vi "Main.vi"() -> ()   [LabVIEW 2020]
panel:
  in  "Test Execution":bool caption="Lab Manager"
  in  "Test Engineering":bool caption="Lab Manager"
  in  "Lab Manager":bool
  # "Please select your operation"
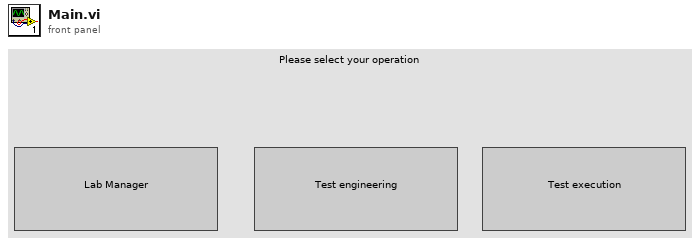
[diagram p1: front panel]
types:
  T1 = enum32{"Invalid", "Standard", "Closed", "Hidden", "Minimized", "Maximized"}
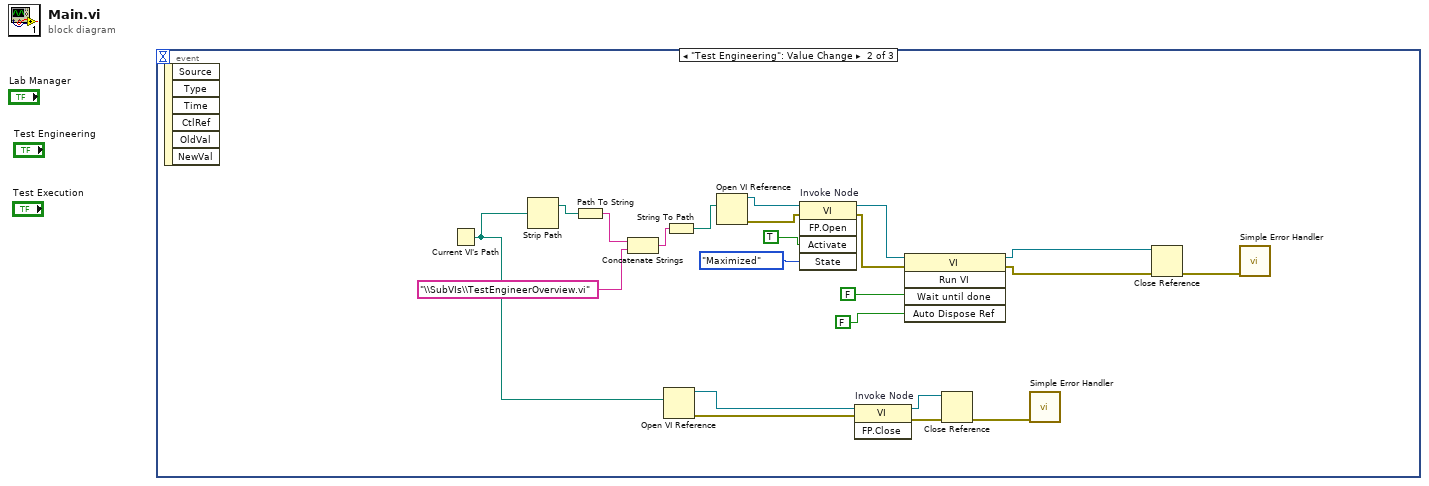
[diagram p0: block diagram]
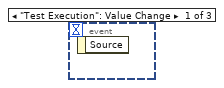
[diagram p2: hidden frame]
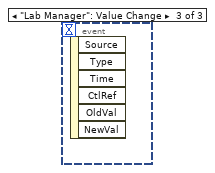
[diagram p3: hidden frame]
diagram:
  n1 = event shown="[1] \"Test Engineering\": Value Change" {
    selector: _ -> [_ _ _]
    dyn-events: _ -> [_ _ _]
    timeout: _ -> [_ _ _]
    event "Test Execution": Value Change {
      n2 = event-data() -> ()  [unwired: 1 in, 1 out]
    }
    event "Test Engineering": Value Change {
      n3 = event-data() -> ()  [unwired: 1 in, 6 out]
      n4 = Current VI's Path() -> (path=w8:path)
      n5 = Strip Path(path=w8) -> (stripped path=w7:path)  [unwired: 1 out]
      n6 = Path To String(path=w7) -> (string=w6:string)
      n7 = Concatenate Strings(w6, "\\SubVIs\\TestEngineerOverview.vi") -> (w4:string)
      n8 = Open VI Reference(vi path=w8) -> (vi reference=w10:refnum<vi>, error out=w9:errorcluster)  [unwired: 5 in]
      n9 = String To Path(string=w4) -> (path=w1:path)
      n10 = Open VI Reference(vi path=w1) -> (vi reference=w3:refnum<vi>, error out=w2:errorcluster)  [unwired: 5 in]
      n11 = invoke on="Invoke Node" class="VI" method="FP.Open"(reference=w3, error in=w2, "Activate"=TRUE ("Activate?"), "State"=T1."Maximized") -> (reference out=w16:refnum<vi>, error out=w17:errorcluster)  [unwired: 1 in, 3 out]
      n12 = invoke on="Invoke Node" class="VI" method="FP.Close"(reference=w10, error in=w9) -> (reference out=w12:refnum<vi>, error out=w13:errorcluster)  [unwired: 1 in, 1 out]
      n13 = invoke class="VI" method="Run VI"(reference=w16, error in=w17, "Wait until done"=FALSE ("Wait Until Done"), "Auto Dispose Ref"=FALSE ("Auto Dispose Reference")) -> (reference out=w15:refnum<vi>, error out=w14:errorcluster)  [unwired: 1 in, 3 out]
      n14 = Close Reference(reference=w12, error in (no error)=w13) -> (error out=w11:errorcluster)
      n15 = call <vilib>:"Simple Error Handler.vi"("error in (no error)"=w11) -> ()  [unwired: 1 in, 8 out]
      n16 = Close Reference(reference=w15, error in (no error)=w14) -> (error out=w22:errorcluster)
      n17 = call <vilib>:"Simple Error Handler.vi"("error in (no error)"=w22) -> ()  [unwired: 1 in, 8 out]
    }
    event "Lab Manager": Value Change {
      n18 = event-data() -> ()  [unwired: 1 in, 6 out]
    }
  }
